vi "Put - NT Enum (Index).vi"(6 "timestamp":timestamp, 7 "PV name":string, 8 "error in (no error)":errorcluster, 9 "timeout":dbl[unit]=1.0, 10 "index":u16, 11 "Client in":refnum<class "Client.lvclass">) -> (0 "error out":errorcluster, 1 "timed out?":bool, 3 "Client out":refnum<class "Client.lvclass">)   [LabVIEW 2020, in "PV Access.lvlib" / "PVA Client.lvlib" / "Client.lvclass"]
uses:
  Client.lvclass
  Client.lvclass/Client.ctl
  PV Data/PV Data/PV Data.lvclass
  PV Data/PV Data/Write Field - I32.vi
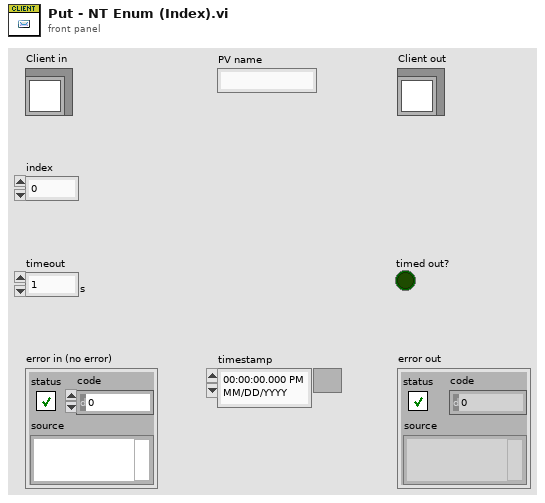
[diagram p1: front panel]
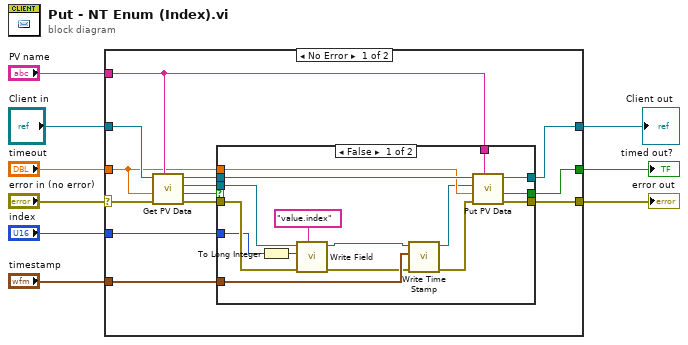
[diagram p0: block diagram]
diagram:
  n1 = case shown="No Error" "error in (no error)" {
    selector: "error in (no error)" -> [w20 w43]
    tunnel: [w19 w43] -> w2
    tunnel: [w18 w42] -> w3
    tunnel: "Client in" -> [w21 w42]
    tunnel: "PV name" -> [w17 _]
    tunnel: "timeout" -> [w15 _]
    tunnel: "index" -> [w10 _]
    tunnel: [w12 _] -> w4
    tunnel: "timestamp" -> [w11 _]
    frame No Error {
      n2 = call "Get PV Data.vi"("PV name"=w17, "error in"=w20, "timeout"=w15, "Client in"=w21) -> ("error out"=w14:errorcluster, "timed out?"=w13:bool, "PV Data out"=w16:refnum<class "PV Data.lvclass">, "Client out"=w22:refnum<class "Client.lvclass">)  [unwired: 4 in]
      n3 = case shown="False" w13 {
        selector: w13 -> [_ w40]
        tunnel: w22 -> [w38 w39]
        tunnel: [w37 w41] -> w19
        tunnel: [w36 w39] -> w18
        tunnel: w17 -> [w35 _]
        tunnel: w16 -> [w34 _]
        tunnel: w15 -> [w33 _]
        tunnel: w14 -> [w32 w41]
        tunnel: [w31 w40] -> w12
        tunnel: w11 -> [w29 _]
        tunnel: w10 -> [w25 _]
        frame False {
          n4 = To Long Integer(number=w25) -> (32bit integer=w26:i32)
          n5 = call-poly "Write Field.vi"("field name"="value.index", "error in"=w32, "value"=w26, "PV Data in"=w34) -> ("error out"=w24:errorcluster, "PV Data out"=w23:refnum<class "PV Data.lvclass">)  [unwired: 5 in, 1 out]
          n6 = call "Write Time Stamp.vi"("error in"=w24, "timestamp in"=w29, "PV Data in"=w23) -> ("error out"=w28:errorcluster, "PV Data out"=w30:refnum<class "PV Data.lvclass">)  [unwired: 5 in, 2 out]
          n7 = call "Put PV Data.vi"("PV name"=w35, "error in"=w28, "timeout"=w33, "PV Data in"=w30, "Client in"=w38) -> ("error out"=w37:errorcluster, "timed out?"=w31:bool, "Client out"=w36:refnum<class "Client.lvclass">)  [unwired: 4 in]
        }
        frame True {
        }
      }
    }
    frame Error {
    }
  }
  "error out" <- w2
  "Client out" <- w3
  "timed out?" <- w4
